vi "joystick_controling_2_robots.vi"() -> ()   [LabVIEW 2016]
uses:
  grSim/grSim Robot Command.ctl
  <vilib>/Instr/_visa.llb/VISA Configure Serial Port (Instr).vi
panel:
  out "String 2":string
  out "Numeric 3":dbl
  out "output cluster 2":T1
  out "string 2":string
  out "return count 2":u32
  out "return count":u32
  in  "stop":bool
  out "string":string
  out "output cluster":T1
  out "String":string
  out "Numeric 2":dbl
  out "error out":errorcluster
  in  "termination char\n(0xA = '\\n' = LF)":u8=10 format="%.0x"
  in  "VISA resource name":refnum<visa-resource-name>
  in  "Serial Settings":T2={"baud rate"=9600, "data bits"=8, "parity"=enum."None", "stop bits"=10, "flow control"=0} {"flow control" items=["None"=0, "XON/XOFF"=1, "RTS/CTS"=2, "DTR/DSR"=4]; "stop bits" items=["1.0"=10, "1.5"=15, "2.0"=20]; "data bits" min=5 max=8 step=1; "baud rate" items=["75"=75, "110"=110, "134"=134, "150"=150, "300"=300, "600"=600, "1200"=1200, "1800"=1800, "2400"=2400, "4800"=4800, "7200"=7200, "9600"=9600, "14400"=14400, "19200"=19200, "28800"=28800, "38400"=38400, "56000"=56000, "57600"=57600, "115200"=115200, "128000"=128000, "230400"=230400]}
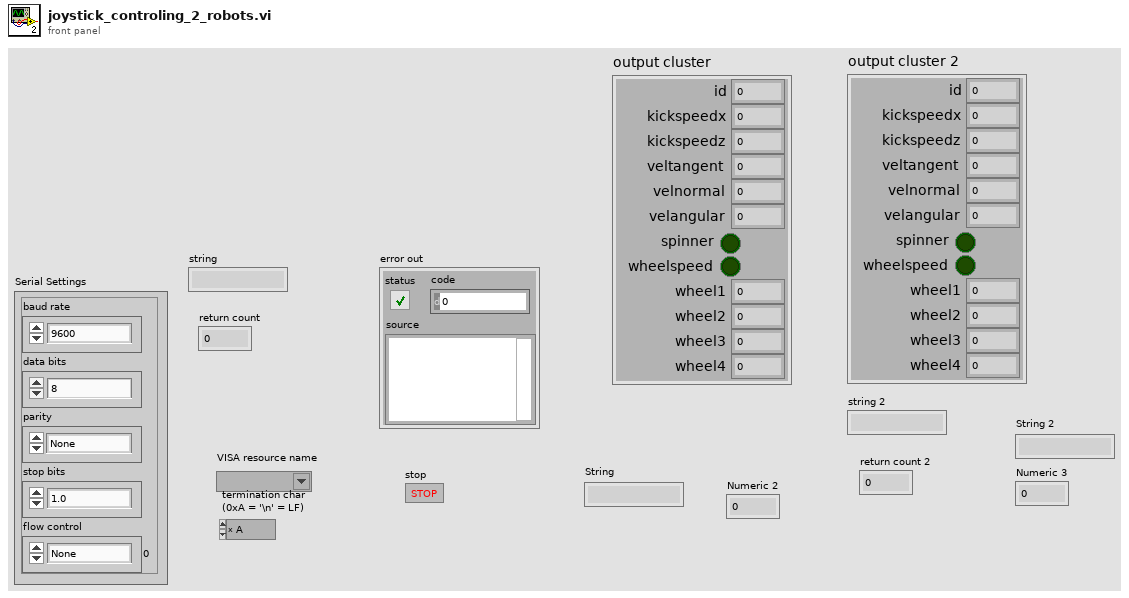
[diagram p1: front panel]
types:
  T1 = typedef "grSim Robot Command.ctl" = cluster{"id":u32, "kickspeedx":sgl, "kickspeedz":sgl, "veltangent":sgl, "velnormal":sgl, "velangular":sgl, "spinner":bool, "wheelspeed":bool, "wheel1":sgl, "wheel2":sgl, "wheel3":sgl, "wheel4":sgl}
  T2 = cluster{"baud rate":u32, "data bits":u16, "parity":enum16{"None", "Odd", "Even", "Mark", "Space"}, "stop bits":u16, "flow control":u16}
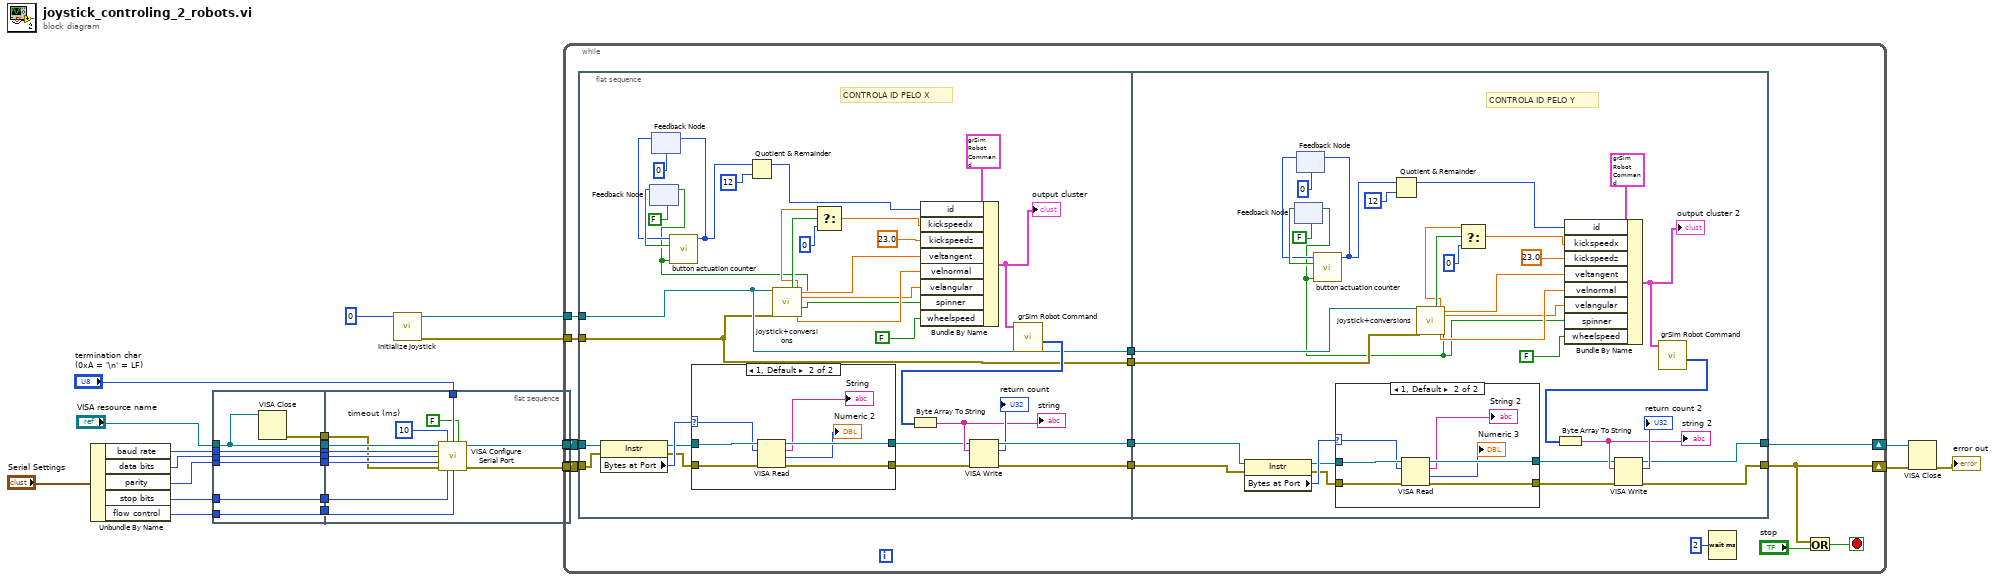
[diagram p0: block diagram]
diagram:
  n1 = Unbundle By Name("Serial Settings") -> ("baud rate"=w15:u32, "data bits"=w14:u16, "parity"=w13:enum16{"None", "Odd", "Even", "Mark", "Space"}, "stop bits"=w12:u16, "flow control"=w11:u16)
  n2 = flat-sequence {
    tunnel: "VISA resource name" -> [w25]
    tunnel: w11 -> [w26]
    tunnel: w12 -> [w27]
    tunnel: w13 -> [w28]
    tunnel: w14 -> [w29]
    tunnel: w15 -> [w30]
    tunnel: [w30] -> w23
    tunnel: [w29] -> w22
    tunnel: [w28] -> w21
    tunnel: [w27] -> w20
    tunnel: [w26] -> w19
    tunnel: [w25] -> w18
    tunnel: [w24] -> w17
    tunnel: "termination char\n(0xA = '\\n' = LF)" -> [w36]
    tunnel: [w34] -> w8
    tunnel: [w33] -> w6
    tunnel: w23 -> [w42]
    tunnel: w22 -> [w41]
    tunnel: w21 -> [w40]
    tunnel: w20 -> [w39]
    tunnel: w19 -> [w38]
    tunnel: w18 -> [w37]
    tunnel: w17 -> [w31]
    frame #0 {
      n3 = VISA Close(VISA resource name=w25) -> (error out=w24:errorcluster)  [unwired: 1 in]
    }
    frame #1 {
      w32 = u32 10  # timeout (ms)
      n4 = call-poly "VISA Configure Serial Port"("VISA resource name"=w37, "timeout (10sec)"=w32, "termination char\n(0xA = '\\n' = LF)"=w36, "Enable Termination\nChar (T)"=FALSE ("Enable Termination\nChar (T)"), "baud rate (9600)"=w42, "data bits (8)"=w41, "parity (0:none)"=w40, "error in (no error)"=w31, "stop bits (10: 1 bit)"=w39, "flow control (0:none)"=w38) -> ("VISA resource name out"=w34:refnum<visa-resource-name>, "error out"=w33:errorcluster)  [unwired: 4 in]
    }
  }
  n5 = call <vilib>:"Initialize Joystick.vi"("device index"=0) -> ("error out"=w1:errorcluster, "device ID"=w2:refnum<k1>)  [unwired: 9 in]
  n6 = while {
    shift-right: [w55] -> w7
    shift-left: w8 -> [w50]
    shift-right: [w44] -> w5
    shift-left: w6 -> [w49]
    tunnel: w2 -> [w52]
    tunnel: w1 -> [w51]
    stop <- w43 stop-if-true
    n7 = flat-sequence {
      tunnel: w52 -> [w58]
      tunnel: w51 -> [w57]
      tunnel: w50 -> [w66]
      tunnel: w49 -> [w65]
      tunnel: [w89] -> w48
      tunnel: [w87] -> w47
      tunnel: [w58] -> w46
      tunnel: [w57] -> w45
      tunnel: [w100] -> w44
      tunnel: [w101] -> w55
      tunnel: w48 -> [w103]
      tunnel: w47 -> [w102]
      tunnel: w46 -> [w105]
      tunnel: w45 -> [w104]
      frame #0 {
        # "CONTROLA ID PELO X"
        n8 = property class="Instr"(reference=w66, error in=w65) -> (reference out=w62:refnum<visa-resource-name>, error out=w63:errorcluster, "Bytes at Port"=w64:u32)
        n9 = feedback #1(FALSE) -> (w76:bool)
        n10 = feedback #2(0) -> (w74:i32)
        n11 = case shown="1, Default" w64 {
          selector: w64 -> [_ w92]
          tunnel: w63 -> [w90 w98]
          tunnel: [w90 w97] -> w68
          tunnel: w62 -> [w91 w96]
          tunnel: [w91 w95] -> w67
          frame 0 {
          }
          frame 1, Default {
            n12 = VISA Read(VISA resource name=w96, byte count=w92, error in (no error)=w98) -> (VISA resource name out=w95:refnum<visa-resource-name>, read buffer=→"String":string, return count=→"Numeric 2":u32, error out=w97:errorcluster)
          }
        }
        n13 = call "joystick+conversions.vi"("Refnum in"=w58, "error in (no error)"=w57) -> ("v_radial"=w80:dbl, "A pressed"=w71:bool, "chute"=w69:dbl, "v_normal"=w82:dbl, "X pressed"=w56:bool, "R*w"=w81:dbl, "Y pressed"=w61:bool)  [unwired: 9 in, 10 out]
        n14 = feedback-in #1(w56) -> ()
        n15 = call "button actuation counter.vi"("old count"=w74, "was button pressed ?"=w76, "button pressed now"=w56) -> ("new count"=w60:i32)  [unwired: 7 in]
        n16 = feedback-in #2(w60) -> ()
        n17 = Quotient & Remainder(x=w60, y=12) -> (x-y*floor(x/y)=w59:i32)  [unwired: 1 out]
        n18 = Select(t=w69, s=w71, f=0) -> (s? t:f=w70:dbl)
        n19 = Bundle By Name(cluster=T1 {"id"=0, "kickspeedx"=0.0, "kickspeedz"=0.0, "veltangent"=0.0, "velnormal"=0.0, "velangular"=0.0, "spinner"=FALSE, "wheelspeed"=FALSE, "wheel1"=0.0, "wheel2"=0.0, "wheel3"=0.0, "wheel4"=0.0} ("Robots"), "id"=w59, "kickspeedx"=w70, "kickspeedz"=sgl 23.0 ("kickspeedx"), "veltangent"=w80, "velnormal"=w82, "velangular"=w81, "spinner"=w61, "wheelspeed"=FALSE) -> (w78:T1)
        "output cluster" <- w78
        n20 = call "grSim Robot Command.vi"("Robots"=w78) -> ("Array"=w85:u8[])  [unwired: 10 in]
        n21 = Byte Array To String(unsigned byte array=w85) -> (string=w86:string)
        "string" <- w86
        n22 = VISA Write(VISA resource name=w67, write buffer=w86, error in (no error)=w68) -> (VISA resource name out=w89:refnum<visa-resource-name>, return count=→"return count":u32, error out=w87:errorcluster)
      }
      frame #1 {
        # "CONTROLA ID PELO Y"
        n23 = property class="Instr"(reference=w103, error in=w102) -> (reference out=w108:refnum<visa-resource-name>, error out=w109:errorcluster, "Bytes at Port"=w110:u32)
        n24 = feedback #3(FALSE) -> (w120:bool)
        n25 = feedback #4(0) -> (w118:i32)
        n26 = case shown="1, Default" w110 {
          selector: w110 -> [_ w134]
          tunnel: w109 -> [w132 w140]
          tunnel: [w132 w139] -> w112
          tunnel: w108 -> [w133 w138]
          tunnel: [w133 w137] -> w111
          frame 0 {
          }
          frame 1, Default {
            n27 = VISA Read(VISA resource name=w138, byte count=w134, error in (no error)=w140) -> (VISA resource name out=w137:refnum<visa-resource-name>, read buffer=→"String 2":string, return count=→"Numeric 3":u32, error out=w139:errorcluster)
          }
        }
        n28 = call "joystick+conversions.vi"("Refnum in"=w105, "error in (no error)"=w104) -> ("v_radial"=w124:dbl, "A pressed"=w115:bool, "chute"=w113:dbl, "v_normal"=w126:dbl, "R*w"=w125:dbl, "Y pressed"=w99:bool)  [unwired: 9 in, 11 out]
        n29 = feedback-in #3(w99) -> ()
        n30 = call "button actuation counter.vi"("old count"=w118, "was button pressed ?"=w120, "button pressed now"=w99) -> ("new count"=w107:i32)  [unwired: 7 in]
        n31 = feedback-in #4(w107) -> ()
        n32 = Quotient & Remainder(x=w107, y=12) -> (x-y*floor(x/y)=w106:i32)  [unwired: 1 out]
        n33 = Select(t=w113, s=w115, f=0) -> (s? t:f=w114:dbl)
        n34 = Bundle By Name(cluster=T1 {"id"=0, "kickspeedx"=0.0, "kickspeedz"=0.0, "veltangent"=0.0, "velnormal"=0.0, "velangular"=0.0, "spinner"=FALSE, "wheelspeed"=FALSE, "wheel1"=0.0, "wheel2"=0.0, "wheel3"=0.0, "wheel4"=0.0} ("Robots"), "id"=w106, "kickspeedx"=w114, "kickspeedz"=sgl 23.0 ("kickspeedx"), "veltangent"=w124, "velnormal"=w126, "velangular"=w125, "spinner"=w99, "wheelspeed"=FALSE) -> (w122:T1)
        "output cluster 2" <- w122
        n35 = call "grSim Robot Command.vi"("Robots"=w122) -> ("Array"=w129:u8[])  [unwired: 10 in]
        n36 = Byte Array To String(unsigned byte array=w129) -> (string=w130:string)
        "string 2" <- w130
        n37 = VISA Write(VISA resource name=w111, write buffer=w130, error in (no error)=w112) -> (VISA resource name out=w101:refnum<visa-resource-name>, return count=→"return count 2":u32, error out=w100:errorcluster)
      }
    }
    n38 = Wait (ms)(milliseconds to wait=u32 2) -> ()  [unwired: 1 out]
    n39 = Or(x=w44, y="stop") -> (x .or. y?=w43:bool)
  }
  n40 = VISA Close(VISA resource name=w7, error in (no error)=w5) -> (error out=→"error out":errorcluster)
